vi "VI Tree.vi"   [LabVIEW 2020, in "BDAQ-6104.lvlib"]
doc: "This is the instrument driver for the <INSTRUMENT NAME>. The VI Tree displays all the user-callable VIs of the instrument driver in an organized table."
uses:
  <instrlib>/BDAQ-6104/BDAQ-6104.lvlib
  <instrlib>/BDAQ-6104/Public/Configure/Configure Edge Counter.vi
  <instrlib>/BDAQ-6104/Public/Data/Read Counter Value.vi
  <instrlib>/BDAQ-6104/Public/Data/Start Streaming.vi
  <instrlib>/BDAQ-6104/Examples/Read Single Digital Channel.vi
  <instrlib>/BDAQ-6104/Public/Data/Read Single Analog Channel.vi
  <instrlib>/BDAQ-6104/Public/Data/Write Single Digital Port.vi
  <instrlib>/BDAQ-6104/Public/Data/Start Counter.vi
panel:
  # "(c) 2014 <Enter Company Name Here>.  ALL RIGHTS RESERVED."
  # "SEE DIAGRAM\nFOR VI TREE."
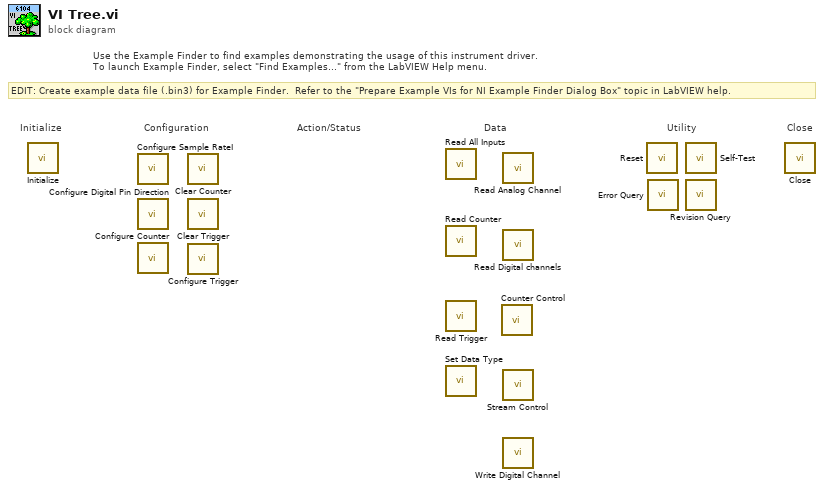
[diagram p0: block diagram]
diagram:
  # "EDIT: Create example data file (.bin3) for Example Finder.  Refer to the \"Prepare Example VIs for NI Example Finder Dialog Box\" topic in LabVIEW help."
  # "Use the Example Finder to find examples demonstrating the usage of this instrument driver.\nTo launch Example Finder, select \"Find Examples...\" from the LabVIEW Help menu."
  # "Configuration"
  # "Utility"
  # "Data"
  # "Action/Status"
  # "Close"
  # "Initialize"
  n1 = call <instrlib>:"Initialize.vi"() -> ()  [unwired: 10 in, 2 out]
  n2 = call <instrlib>:"Configure Sample RateI.vi"() -> ()  [unwired: 10 in, 2 out]
  n3 = call <instrlib>:"Configure Digital Pin Direction.vi"() -> ()  [unwired: 10 in, 2 out]
  n4 = call-poly <instrlib>:"Configure Counter.vi"() -> ()  [unwired: 10 in, 2 out]
  n5 = call <instrlib>:"Clear Counter.vi"() -> ()  [unwired: 10 in, 2 out]
  n6 = call <instrlib>:"Clear Trigger.vi"() -> ()  [unwired: 10 in, 2 out]
  n7 = call <instrlib>:"Configure Trigger.vi"() -> ()  [unwired: 10 in, 2 out]
  n8 = call <instrlib>:"Read All Inputs.vi"() -> ()  [unwired: 8 in, 4 out]
  n9 = call-poly <instrlib>:"Read Counter.vi"() -> ()  [unwired: 9 in, 3 out]
  n10 = call <instrlib>:"Read Trigger.vi"() -> ()  [unwired: 9 in, 3 out]
  n11 = call <instrlib>:"Set Data Type.vi"() -> ()  [unwired: 10 in, 2 out]
  n12 = call-poly <instrlib>:"Counter Control.vi"() -> ()  [unwired: 10 in, 2 out]
  n13 = call-poly <instrlib>:"Read Analog Channel.vi"() -> ()  [unwired: 9 in, 3 out]
  n14 = call-poly <instrlib>:"Read Digital channels.vi"() -> ()  [unwired: 9 in, 3 out]
  n15 = call-poly <instrlib>:"Stream Control.vi"() -> ()  [unwired: 10 in, 2 out]
  n16 = call-poly <instrlib>:"Write Digital Channel.vi"() -> ()  [unwired: 10 in, 2 out]
  n17 = call <instrlib>:"Reset.vi"() -> ()  [unwired: 10 in, 2 out]
  n18 = call <instrlib>:"Error Query.vi"() -> ()  [unwired: 8 in, 4 out]
  n19 = call <instrlib>:"Self-Test.vi"() -> ()  [unwired: 8 in, 4 out]
  n20 = call <instrlib>:"Revision Query.vi"() -> ()  [unwired: 8 in, 4 out]
  n21 = call <instrlib>:"Close.vi"() -> ()  [unwired: 11 in, 1 out]
